vi "TypeCodeToEnum.vi"(11 "Type Code (numbers in hexadecimal)":i16 format="%.0x") -> (2 "UDV Data Type":string, 3 "UDV Data Type":T1)   [LabVIEW 2017, in "Scan Engine Custom Device.lvlib"]
uses:
  Scan Engine Custom Device.lvlib
  Type Defs/ECAT Channel Data Type.ctl
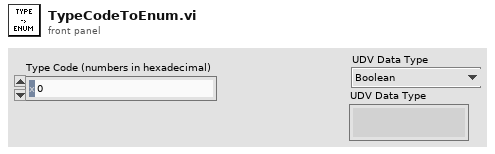
[diagram p1: front panel]
types:
  T1 = typedef "Scan Engine Custom Device.lvlib/ECAT Channel Data Type.ctl" = enum16{"Boolean", "Fixed Point", "Int8", "Int16", "Int32", "Int64", "U32 Bit Field", "UInt8", "UInt16", "UInt32", "UInt64", "Other", "DBL", "SGL"}
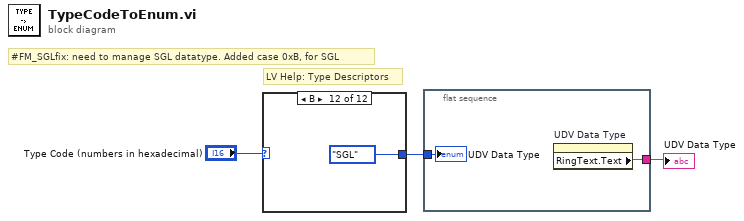
[diagram p0: block diagram]
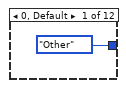
[diagram p2: hidden frame]
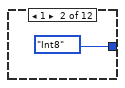
[diagram p3: hidden frame]
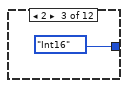
[diagram p4: hidden frame]
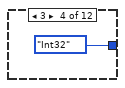
[diagram p5: hidden frame]
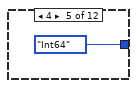
[diagram p6: hidden frame]
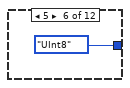
[diagram p7: hidden frame]
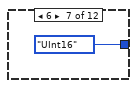
[diagram p8: hidden frame]
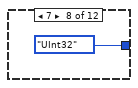
[diagram p9: hidden frame]
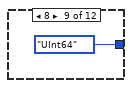
[diagram p10: hidden frame]
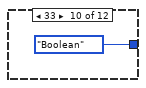
[diagram p11: hidden frame]
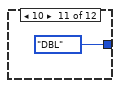
[diagram p12: hidden frame]
diagram:
  # "#FM_SGLfix: need to manage SGL datatype. Added case 0xB, for SGL"
  # "LV Help: Type Descriptors"
  n1 = case shown="B" "Type Code (numbers in hexadecimal)" {
    tunnel: [ECAT_Channel_Data_Type."Other" ("UDV Data Type") ECAT_Channel_Data_Type."Int8" ("UDV Data Type") ECAT_Channel_Data_Type."Int16" ("UDV Data Type") ECAT_Channel_Data_Type."Int32" ("UDV Data Type") ECAT_Channel_Data_Type."Int64" ("UDV Data Type") ECAT_Channel_Data_Type."UInt8" ("UDV Data Type") ECAT_Channel_Data_Type."UInt16" ("UDV Data Type") ECAT_Channel_Data_Type."UInt32" ("UDV Data Type") ECAT_Channel_Data_Type."UInt64" ("UDV Data Type") ECAT_Channel_Data_Type."Boolean" ("UDV Data Type") ECAT_Channel_Data_Type."DBL" ("UDV Data Type") ECAT_Channel_Data_Type."SGL" ("UDV Data Type")] -> w2
    frame 0, Default {
    }
    frame 1 {
    }
    frame 2 {
    }
    frame 3 {
    }
    frame 4 {
    }
    frame 5 {
    }
    frame 6 {
    }
    frame 7 {
    }
    frame 8 {
    }
    frame 33 {
    }
    frame 10 {
    }
    frame 11 {
    }
  }
  n2 = flat-sequence {
    tunnel: w2 -> [w17]
    tunnel: [w16] -> w1
    frame #0 {
      n3 = property on="UDV Data Type" class="Enum (strict)"() -> ("RingText.Text"=w16:string)  [unwired: 2 in, 2 out]
      "UDV Data Type" <- w17
    }
  }
  "UDV Data Type" <- w1
